vi "ad get next run f64.vi"(7 "p":dbl[](array[numeric]), 8 "error in (no error)":errorcluster, 9 "run":u32, 10 "state":T1, 11 "adh":i32) -> (0 "error out":errorcluster, 1 "run out":u32, 2 "state out":T1, 3 "function return":i32, 5 "p out":dbl[](array[numeric]))   [LabVIEW 2021, in "libad4.lvlib"]
doc: "LIBAD4 function: ad_get_next_run_f64 (int32_t adh, struct ad_scan_state *state, uint32_t *run, double *p);\n\nReturns the measurements from a scan run. Returns measurements and converts to float representation.\nf64 version required for 32bit DAQs."
uses:
  <userlib>/libad4/libad4.lvlib
  <userlib>/libad4/controls/ad scan state.ctl
  <userlib>/libad4/libad4.dll
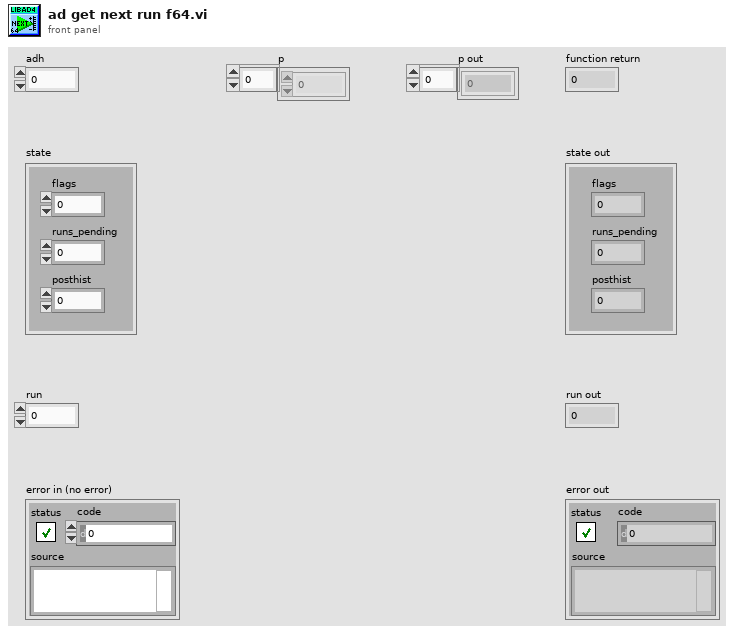
[diagram p1: front panel]
types:
  T1 = typedef "libad4.lvlib/ad scan state.ctl" = cluster{"flags":i32, "runs_pending":i32, "posthist":i64}
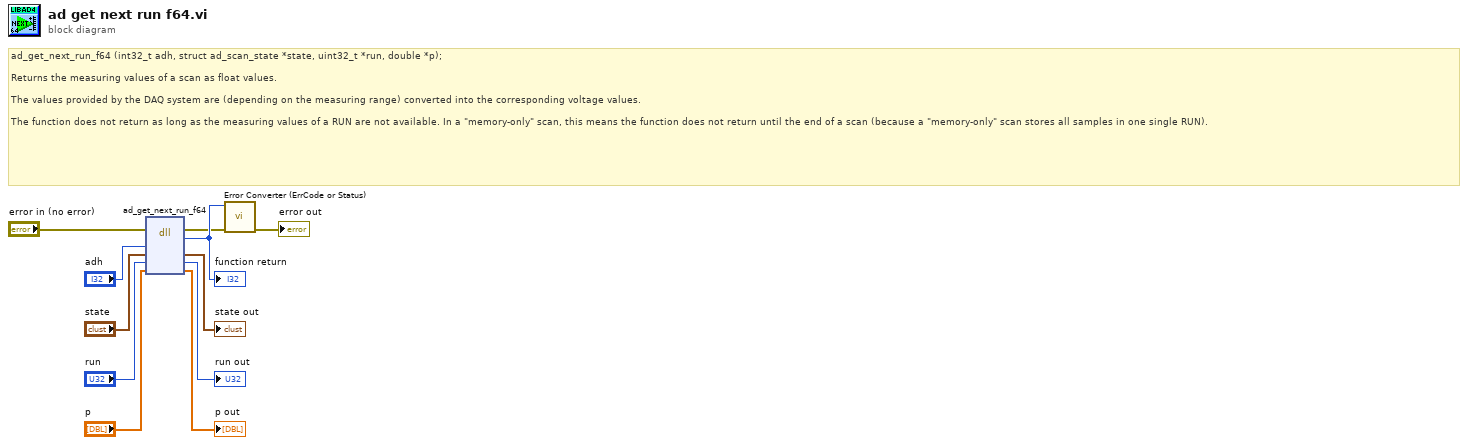
[diagram p0: block diagram]
diagram:
  # "ad_get_next_run_f64 (int32_t adh, struct ad_scan_state *state, uint32_t *run, double *p);\n\nReturns the measuring values of a scan as float values.\n\nThe values provided by the DAQ system are (depending on the measuring range) converted into the corresponding voltage values.\n\nThe function does not return as long as the measuring values of a RUN are not available. In a \"memory-only\" scan, this means the function does not return until the end of a scan (because a \"memory-only\" scan stores all samples in one single RUN)."
  n1 = dll-call lib="C:/Program Files/National Instruments/LabVIEW 2021/user.lib/libad4/libad4.*" fn="ad_get_next_run_f64"(error in="error in (no error)", "adh"="adh", "state"="state", "run"="run", "p"="p") -> (error out=w2:errorcluster, "return type"=w11:i32, "state"=→"state out":T1, "run"=→"run out":u32, "p"=→"p out":dbl[])  [unwired: 3 in, 1 out]
  "function return" <- w11
  n2 = call <userlib>:"Error Converter (ErrCode or Status).vi"("error in (no error)"=w2, "error code"=w11) -> ("error out"=→"error out":errorcluster)  [unwired: 9 in]
